vi "camera defaults globals.vi"() -> ()   [LabVIEW 2015]
uses:
  ixon camera/image size.ctl
panel:
  in  "Image Size Limits":T1={"H Bin"=1, "V Bin"=1, "Left"=1, "Top"=1, "Right"=1024, "Bottom"=1024}
  in  "Default Image Size":T1={"H Bin"=1, "V Bin"=1, "Left"=1, "Top"=276, "Right"=1024, "Bottom"=815}
  # "iXon Ultra 1024"
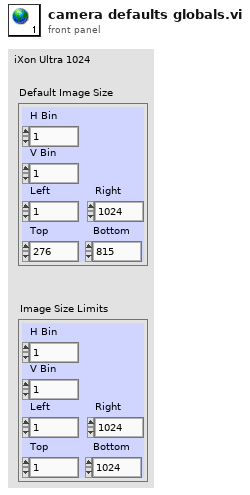
[diagram p1: front panel]
types:
  T1 = typedef "image size.ctl" = cluster{"H Bin":i32, "V Bin":i32, "Left":i32, "Top":i32, "Right":i32, "Bottom":i32}
diagram:
